vi "Update Cal Config File from GU Bench.vi"(7 "Output File Path":path, 8 "error in":errorcluster, 10 "GU Bench File Path":path, 11 "Calibration Config File Path":path) -> (0 "error out":errorcluster)   [LabVIEW 2020, in "GUCalibration2.lvlib"]
uses:
  GUCalibration2.lvlib
  <vilib>/Utility/file.llb/Write Delimited Spreadsheet (string).vi
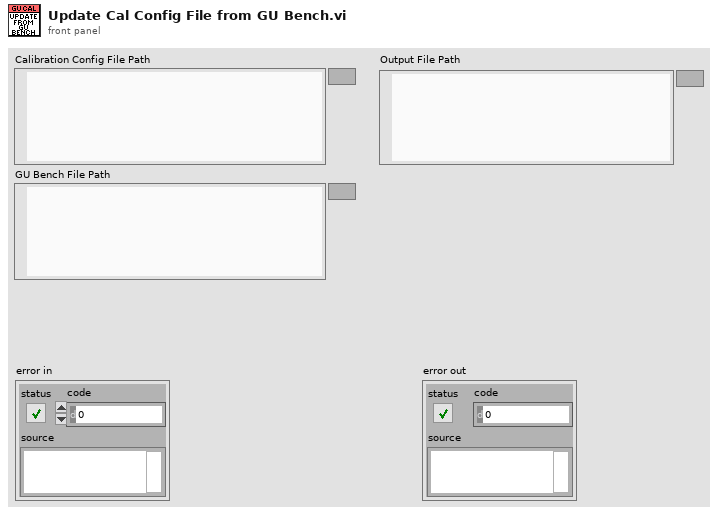
[diagram p1: front panel]
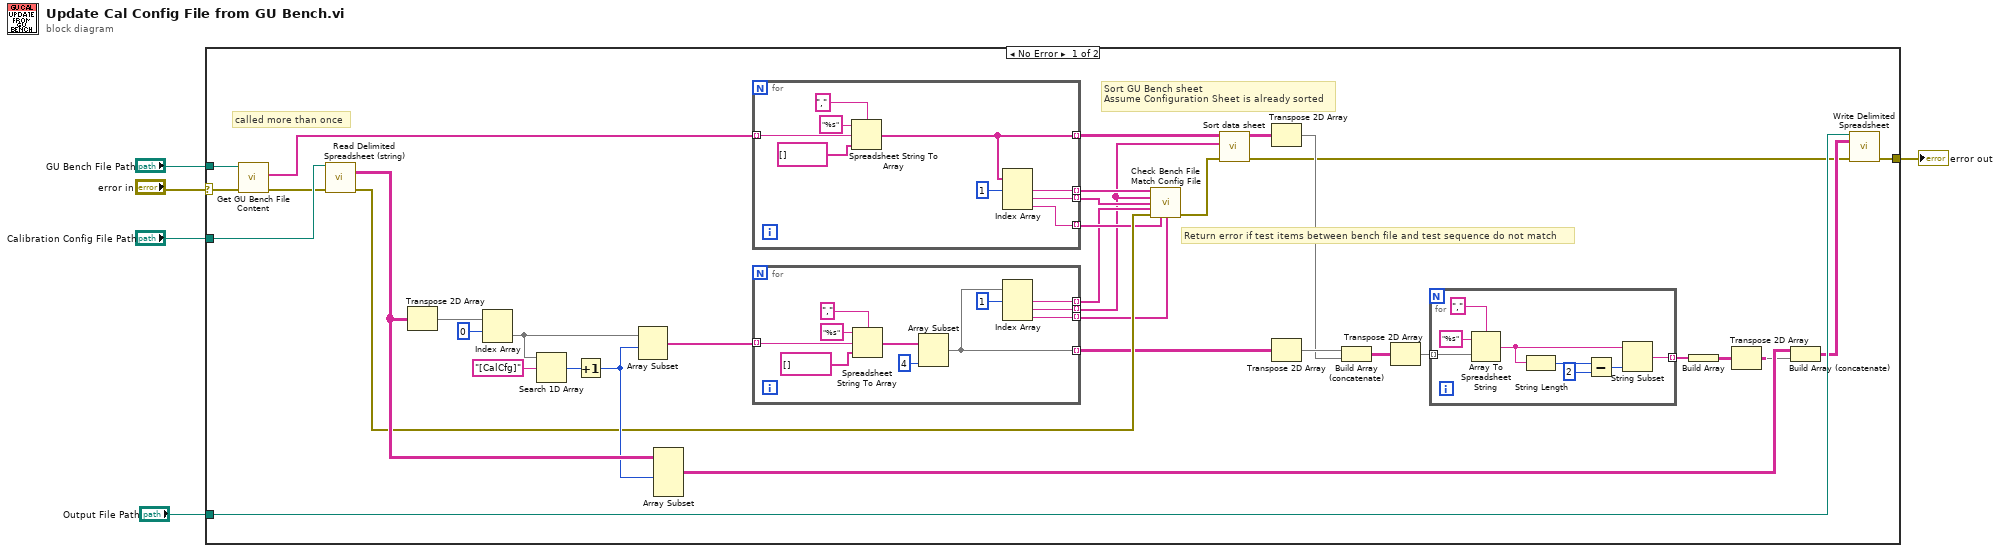
[diagram p0: block diagram]
diagram:
  n1 = case shown="No Error" "error in" {
    selector: "error in" -> [w12 w70]
    tunnel: "Calibration Config File Path" -> [w36 _]
    tunnel: "Output File Path" -> [w24 _]
    tunnel: [w22 w70] -> w3
    tunnel: "GU Bench File Path" -> [w16 _]
    frame No Error {
      # "called more than once"
      # "Return error if test items between bench file and test sequence do not match"
      # "Sort GU Bench sheet\nAssume Configuration Sheet is already sorted"
      n2 = call "Get GU Bench File Content.vi"("error in"=w12, "GU Bench File Path"=w16) -> ("error out"=w14:errorcluster, "Get GU Bench Content"=w15:string[])  [unwired: 8 in]
      n3 = call <vilib>:"Read Delimited Spreadsheet (string).vi"("file path (dialog if empty)"=w36, "error in (no error)"=w14) -> ("all rows"=w31:string[][], "error out"=w20:errorcluster)  [unwired: 8 in, 4 out]
      n4 = Transpose 2D Array(2D array=w31) -> (transposed array=w40:string[][])
      n5 = Index Array(array=w40, index (row)=0) -> (element=w37:string[])  [unwired: 1 in]
      n6 = Search 1D Array(1D array=w37, element="[CalCfg]") -> (index of element=w38:i32)  [unwired: 1 in]
      n7 = Increment(x=w38) -> (x+1=w30:i32)
      n8 = Array Subset(array=w37, index=w30) -> (w10:string[])  [unwired: 1 in]
      n9 = Array Subset(array=w31, length (row)=w30) -> (w26:string[][])  [unwired: 3 in]
      n10 = for {
        tunnel: w15 -> [w66] mode=indexing
        tunnel: [w63] -> w19 mode=indexing
        tunnel: [w65] -> w35 mode=indexing
        tunnel: [w62] -> w18 mode=indexing
        tunnel: [w61] -> w11 mode=indexing
        n11 = Spreadsheet String To Array(delimiter (Tab)=",", format string="%s", spreadsheet string=w66, array type (2D Dbl)=string[] []) -> (array=w65:string[])
        n12 = Index Array(array=w65, index #1=1 ("index")) -> (element #1=w63:string, element #2=w62:string, element #3=w61:string)  [unwired: 2 in]
      }
      n13 = for {
        tunnel: w10 -> [w47] mode=indexing
        tunnel: [w45] -> w8 mode=indexing
        tunnel: [w44] -> w6 mode=indexing
        tunnel: [w43] -> w7 mode=indexing
        tunnel: [w42] -> w9 mode=indexing
        n14 = Spreadsheet String To Array(delimiter (Tab)=",", format string="%s", spreadsheet string=w47, array type (2D Dbl)=string[] []) -> (array=w51:string[])
        n15 = Array Subset(array=w51, length=4 ("index")) -> (w45:string[])  [unwired: 1 in]
        n16 = Index Array(array=w45, index #1=1 ("index")) -> (element #1=w43:string, element #2=w44:string, element #3=w42:string)  [unwired: 2 in]
      }
      n17 = call "Check Bench File Match Config File.vi"("Bench File Test Number"=w19, "Config File Test Number"=w6, "Bench File Test Name"=w18, "Config File Test Name"=w7, "error in"=w20, "Bench File Test Unit"=w11, "Config File Test Unit"=w9) -> ("error out"=w21:errorcluster)  [unwired: 8 in]
      n18 = call "Sort data sheet.vi"("error in"=w21, "Config File Test Number"=w6, "Input Data Sheet"=w35) -> ("error out"=w13:errorcluster, "Output Data Sheet"=w17:string[][])  [unwired: 7 in]
      n19 = Transpose 2D Array(2D array=w17) -> (transposed array=w33:string[][])
      n20 = Transpose 2D Array(2D array=w8) -> (transposed array=w34:string[][])
      n21 = Build Array (concatenate)(w34, w33) -> (w32:string[][])
      n22 = Transpose 2D Array(2D array=w32) -> (transposed array=w29:string[][])
      n23 = for {
        tunnel: w29 -> [w58] mode=indexing
        tunnel: [w53] -> w28 mode=indexing
        n24 = Array To Spreadsheet String(delimiter (Tab)=",", array=w58, 3:"%s" ("format string")) -> (spreadsheet string=w54:string)
        n25 = String Length(string=w54) -> (length=w57:i32)
        n26 = Subtract(x=w57, y=2) -> (x-y=w55:i32)
        n27 = String Subset(string=w54, length (rest)=w55) -> (substring=w53:string)  [unwired: 1 in]
      }
      n28 = Build Array(w28) -> (w27:string[][])
      n29 = Transpose 2D Array(2D array=w27) -> (transposed array=w25:string[][])
      n30 = Build Array (concatenate)(w26, w25) -> (w23:string[][])
      n31 = call-poly <vilib>:"Write Delimited Spreadsheet.vi"("file path (dialog if empty)"=w24, "2D data"=w23, "error in (no error)"=w13) -> ("error out"=w22:errorcluster)  [unwired: 11 in, 1 out]
    }
    frame Error {
    }
  }
  "error out" <- w3
